vi "init.vi"(8 "error in (no error)":errorcluster, 10 "Init Data":variant, 11 "Lesker Pressure in":refnum<class "Lesker Pressure.lvclass">) -> (0 "error out":errorcluster, 2 "Channel List":refnum<class "HK Item.lvclass">[](array[class]), 3 "Lesker Pressure out":refnum<class "Lesker Pressure.lvclass">)   [LabVIEW 2021, in "Lesker Pressure.lvclass"]
uses:
  Lesker Pressure.lvclass
  hk-channel-class/HK Item/HK Item.lvclass
  CC cluster Pressure Monitor Settings.ctl
  Lesker Pressure.lvclass/Lesker Pressure.ctl
  Pressure Monitor.lvclass
panel:
  # "LESKER 392 Series"
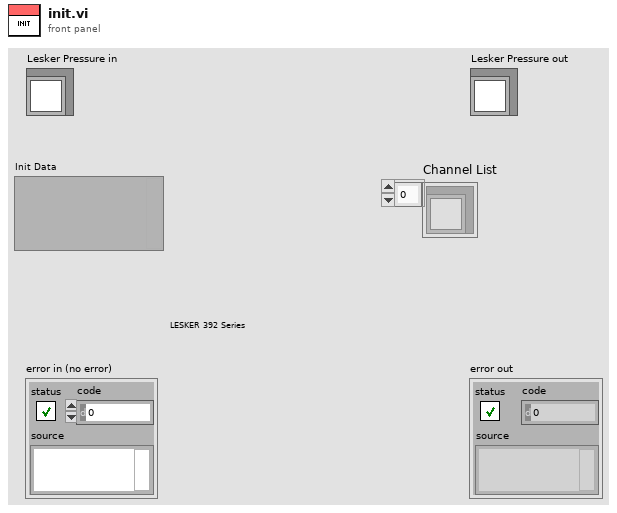
[diagram p1: front panel]
types:
  T1 = typedef "CC cluster Pressure Monitor Settings.ctl" = cluster{"Lesker Addrs":refnum<visa-resource-name>[], "Enabled?":bool[], "Pressure Alarm Level":dbl, "Filaments":bool[]}
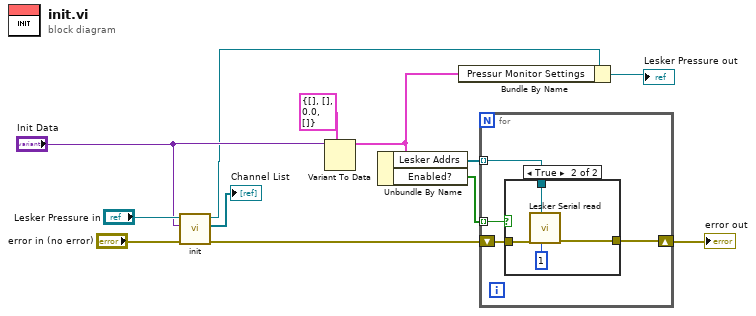
[diagram p0: block diagram]
diagram:
  n1 = call-parent "init.vi"("error in (no error)"="error in (no error)", "Init Data"="Init Data", "Pressure Monitor in"="Lesker Pressure in") -> ("error out"=w9:errorcluster, "Channel List"=→"Channel List":refnum<class "HK Item.lvclass">[], "Pressure Monitor out"=w5:refnum<class "Lesker Pressure.lvclass">)  [unwired: 6 in]
  n2 = Variant To Data(type=T1 {"Lesker Addrs"=[], "Enabled?"=[], "Pressure Alarm Level"=0.0, "Filaments"=[]} ("Pressur Monitor Settings"), Variant="Init Data") -> (data=w2:T1)  [unwired: 1 in, 1 out]
  n3 = Unbundle By Name(w2) -> ("Lesker Addrs"=w4:refnum<visa-resource-name>[], "Enabled?"=w1:bool[])
  n4 = Bundle By Name(cluster=w5, "Pressur Monitor Settings"=w2) -> (→"Lesker Pressure out":refnum<class "Lesker Pressure.lvclass">)
  n5 = for {
    tunnel: w4 -> [w16] mode=indexing
    shift-right: [w14] -> w8
    shift-left: w9 -> [w15]
    tunnel: w1 -> [w13] mode=indexing
    n6 = case shown="True" w13 {
      tunnel: w16 -> [_ w21]
      tunnel: w15 -> [w17 w20]
      tunnel: [w17 w19] -> w14
      frame False {
      }
      frame True {
        n7 = call "Lesker Serial read.vi"("Number of reads"=1, "VISA resource name"=w21, "error in (no error)"=w20) -> ("error out"=w19:errorcluster)  [unwired: 6 in, 2 out]
      }
    }
  }
  "error out" <- w8
